vi "Procesado_aRMS_BIdirecc.vi"(0 "Paths_canales_aRMS":path[](array[path]), 3 "Ejes Procesados":i32, 4 "Distancias\nacelerometros":dbl[](array[numeric]), 6 "Distancias generales (m)":dbl[](array[numeric]), 7 "Distancias centrales de las ruedas\n               configuración (m)":dbl[](array[numeric]), 8 "Frecuencia de muestreo":dbl, 9 "Parámetros acelerómetros":dbl[](array[numeric]), 10 "dt RMS 2":dbl, 11 "Puntos":sgl[](array[numeric])) -> (1 "Max RMS Ruedas":dbl[][](array[numeric]))   [LabVIEW 2015]
uses:
  <vilib>/Analysis/3filter.llb/Filter Passband Type.ctl
  <vilib>/Analysis/5stat.llb/RMS (DBL).vi
  <vilib>/Analysis/3filter.llb/Butterworth Filter (DBL).vi
  <vilib>/measure/madcrms.llb/Basic Averaged DC-RMS for 1 Chan.vi
  <vilib>/measure/NI_MAPro.lvlib
  <vilib>/Analysis/NI_AALBase.lvlib
  <vilib>/Analysis/NI_AALPro.lvlib
panel:
  out "Array 2":dbl[][](array[numeric])
  out "Array":dbl[][](array[numeric])
  out "Loop Rate (Hz)":dbl
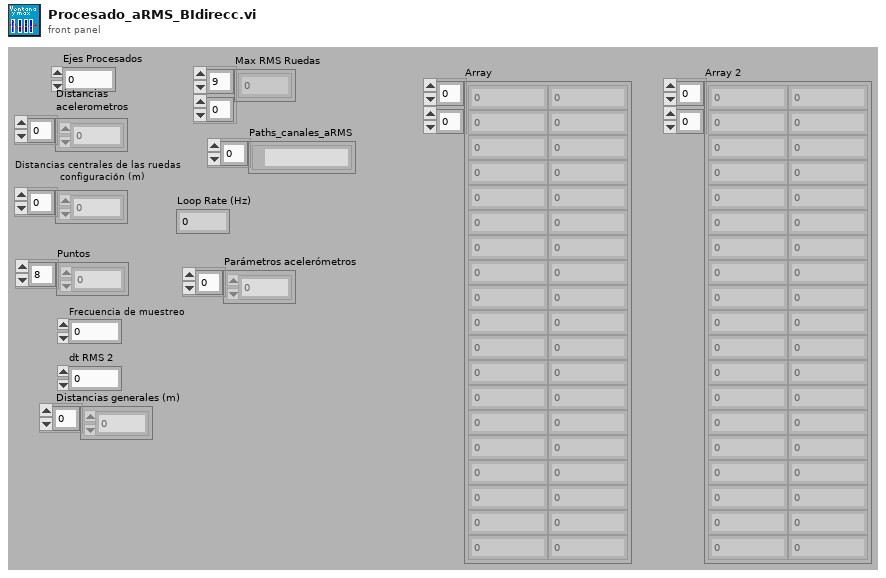
[diagram p1: front panel]
types:
  T1 = typedef "NI_AALBase.lvlib/Filter Passband Type.ctl" = enum32{"Lowpass", "Highpass", "Bandpass", "Bandstop"}
  T2 = enum16{"big-endian, network order", "native, host order", "little-endian"}
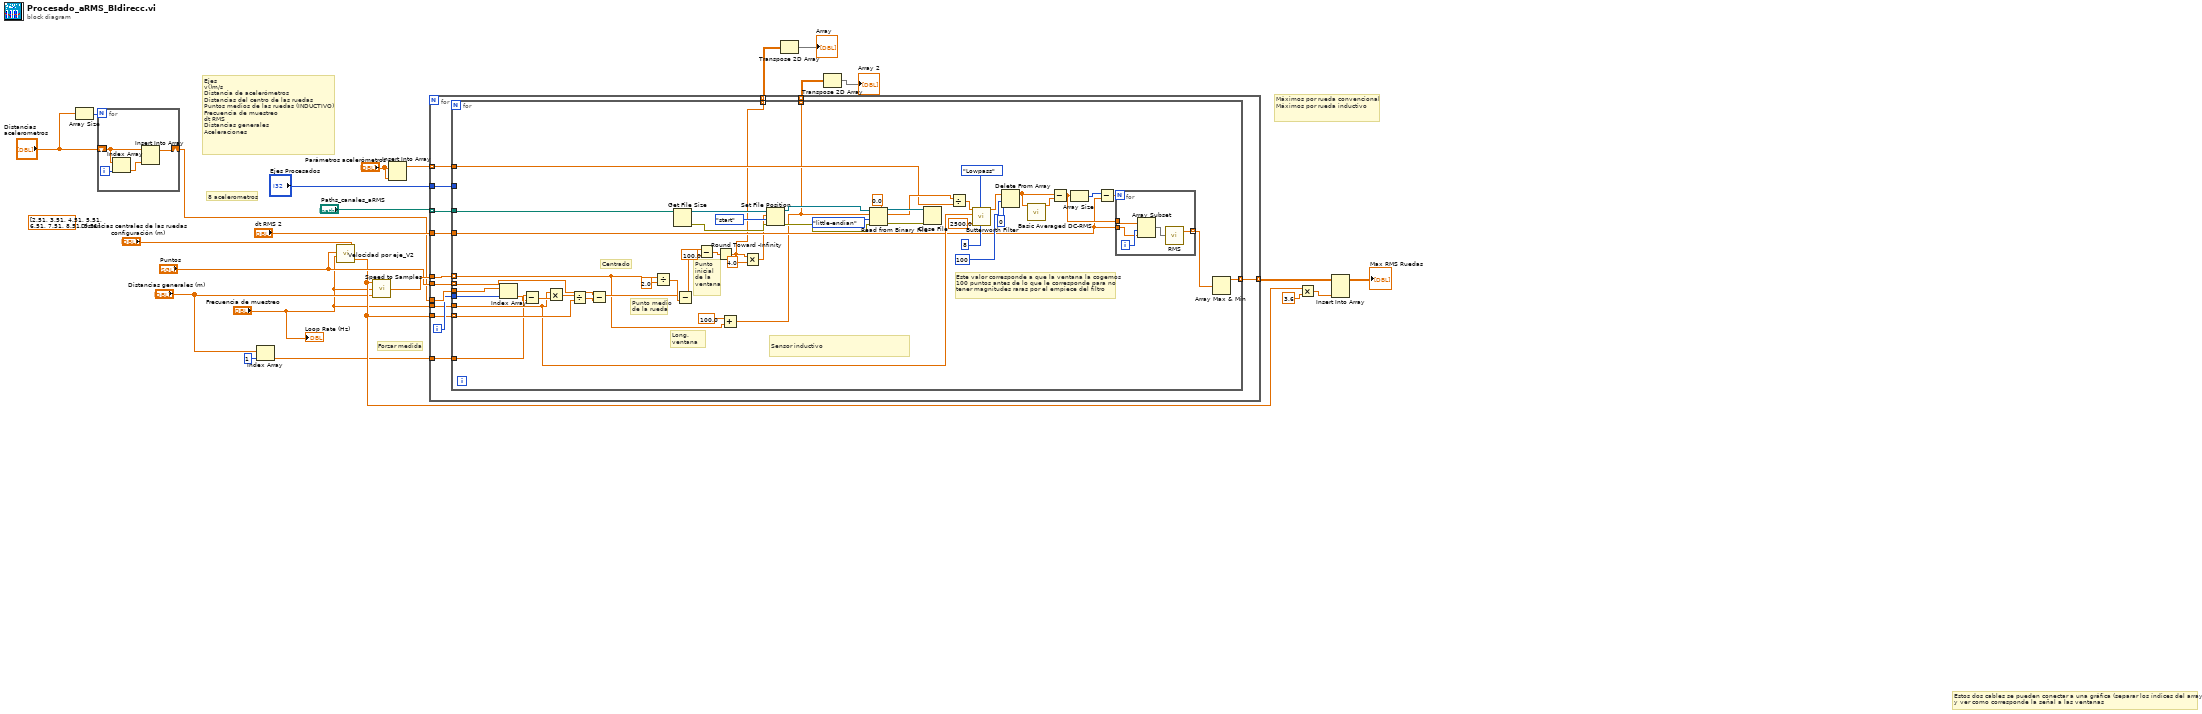
[diagram p0: block diagram]
diagram:
  (unwired) dbl[] [2.51, 3.51, 4.51, 5.51, 6.51, 7.51, 8.51, 9.51] ("Distancias\nacelerometros")
  # "Forzar medida"
  # "8 acelerometros"
  # "Ejes\nv()m/s\nDistancia de acelerómetros\nDistancias del centro de las ruedas\nPuntos medios de las ruedas (INDUCTIVO)\nFrecuencia de muestreo\ndt RMS\nDistancias generales\nAceleraciones"
  # "Máximos por rueda convencional\nMáximos por rueda inductivo"
  # "Estos dos cables se pueden conectar a una gráfica (separar los índices del array)\ny ver como corresponde la señal a las ventanas"
  n1 = Array Size(array="Distancias\nacelerometros") -> (size(s)=w8:i32)
  n2 = for {
    N: w8 -> [_]
    shift-right: [w28] -> w2
    shift-left: "Distancias\nacelerometros" -> [w27]
    i -> [w26]
    n3 = Index Array(array=w27, index=w26) -> (element=w25:dbl)
    n4 = Insert Into Array(array=w27, new element=w25) -> (w28:dbl[])  [unwired: 1 in]
  }
  n5 = Index Array(array="Distancias generales (m)", index=1) -> (element=w1:dbl)
  n6 = call "Velocidad por eje_V2.vi"("Distancias centrales de las ruedas\n               configuración (m)"="Distancias centrales de las ruedas\n               configuración (m)", "Frecuencia de muestreo"="Frecuencia de muestreo", "Puntos centrales de las ruedas\n             inductivo"="Puntos") -> ("Velocidad de eje"=w18:dbl[])  [unwired: 2 in]
  n7 = call "Speed to Samples.vi"("Distancias generales (m)"="Distancias generales (m)", "Loop Rate (Hz)"="Frecuencia de muestreo", "Velocidad de eje(m/s)"=w18) -> ("Longitud de ventana (puntos)"=w24:dbl[])
  n8 = Insert Into Array(array="Parámetros acelerómetros", new element="Parámetros acelerómetros") -> (w13:dbl[])  [unwired: 1 in]
  n9 = for {
    tunnel: w24 -> [w32]
    tunnel: "Puntos" -> [w40]
    tunnel: w18 -> [w37]
    tunnel: w2 -> [w41]
    tunnel: "dt RMS 2" -> [w42]
    tunnel: [w39] -> w20 mode=indexing
    tunnel: "Ejes Procesados" -> [w33]
    tunnel: "Frecuencia de muestreo" -> [w34]
    tunnel: "Paths_canales_aRMS" -> [w36] mode=indexing
    tunnel: w13 -> [w35] mode=indexing
    tunnel: w1 -> [w31]
    tunnel: [w30] -> w3 mode=indexing
    tunnel: [w29] -> w6 mode=indexing
    i -> [w38]
    n10 = for {
      tunnel: w42 -> [w49]
      tunnel: w41 -> [w90]
      tunnel: w40 -> [w89] mode=indexing
      tunnel: [w88] -> w39 mode=indexing
      tunnel: w38 -> [w87]
      tunnel: w37 -> [w86] mode=indexing
      tunnel: w36 -> [w71]
      tunnel: w35 -> [w80]
      tunnel: w34 -> [w63]
      tunnel: w33 -> [_]
      tunnel: w32 -> [w60] mode=indexing
      tunnel: w31 -> [w47]
      tunnel: [w44] -> w30 mode=indexing
      tunnel: [w43] -> w29 mode=indexing
      # "Este valor corresponde a que la ventana la cogemos\n100 puntos antes de lo que le corresponde para no \ntener magnitudes raras por el empiece del filtro"
      # "Centrado"
      # "Sensor inductivo"
      # "Long.\nventana"
      # "Punto\ninicial\nde la \nventana"
      # "Punto medio\nde la rueda"
      n11 = Index Array(array=w90, index=w87) -> (element=w46:dbl)
      n12 = Subtract(x=w47, y=w46) -> (x-y=w74:dbl)
      n13 = Multiply(x=w63, y=w74) -> (x*y=w76:dbl)
      n14 = Divide(x=w76, y=w86) -> (x/y=w75:dbl)
      n15 = Subtract(x=w89, y=w75) -> (x-y=w64:dbl)
      n16 = Divide(x=w60, y=2.0) -> (x/y=w72:dbl)
      n17 = Get File Size(file=w71) -> (refnum out=w69:refnum<file>, 0:w66:errorcluster)  [unwired: 1 in, 1 out]
      n18 = Subtract(x=w64, y=w72) -> (x-y=w54:dbl)
      n19 = Subtract(x=w54, y=100.0 ("x")) -> (x-y=w62:dbl)
      n20 = Round Toward -Infinity(1:w62) -> (0:w44:dbl)
      n21 = Add(x=100.0, y=w60) -> (x+y=w43:dbl)
      n22 = Multiply(x=w44, y=4.0) -> (x*y=w45:dbl)
      n23 = Set File Position(offset (in bytes) (0)=w45, refnum=w69, from (0:start)=enum16{"start", "end", "current"}."start", error in=w66) -> (refnum out=w67:refnum<file>, error out=w65:errorcluster)
      n24 = Read from Binary File(5:sgl 0.0, 8:w65, 9:T2."little-endian" ("byte order (0:big-endian, network order)"), 10:w43, 11:w67) -> (0:w84:errorcluster, 2:w81:sgl[], 3:w85:refnum<file>)  [unwired: 2 out]
      n25 = Close File(refnum=w85, error in=w84) -> ()  [unwired: 2 out]
      n26 = Divide(x=w81, y=w80) -> (x/y=w77:dbl[])
      n27 = call-poly <vilib>:"Butterworth Filter.vi"("order"=8, "filter type"=Filter_Passband_Type."Lowpass", "low cutoff freq: fl"=2500.0, "sampling freq: fs"=w63, "X"=w77) -> ("Filtered X"=w59:dbl[])  [unwired: 3 in, 1 out]
      n28 = Delete From Array(array=w59, length=100, index=0) -> (array with subset deleted=w58:dbl[])  [unwired: 1 out]
      n29 = call-poly <vilib>:"Basic Averaged DC-RMS.vi"("signal in"=w58) -> ("DC value"=w91:dbl)  [unwired: 4 in, 6 out]
      n30 = Subtract(x=w58, y=w91) -> (x-y=w52:dbl[])
      n31 = Array Size(array=w52) -> (size(s)=w50:i32)
      n32 = Subtract(x=w50, y=w49) -> (x-y=w51:dbl)
      n33 = for {
        N: w51 -> [_]
        tunnel: w49 -> [w93]
        tunnel: [w96] -> w48 mode=indexing
        tunnel: w52 -> [w95]
        i -> [w94]
        n34 = Array Subset(array=w95, index=w94, length=w93) -> (w92:dbl[])
        n35 = call-poly <vilib>:"RMS.vi"("X"=w92) -> ("rms value"=w96:dbl)  [unwired: 1 out]
      }
      n36 = Array Max & Min(array=w48) -> (max value=w88:dbl)  [unwired: 3 out]
    }
  }
  n37 = Transpose 2D Array(2D array=w3) -> (transposed array=→"Array":dbl[][])
  n38 = Transpose 2D Array(2D array=w6) -> (transposed array=→"Array 2":dbl[][])
  n39 = Multiply(x=w18, y=3.6) -> (x*y=w16:dbl[])
  n40 = Insert Into Array(array=w20, new element=w16) -> (→"Max RMS Ruedas":dbl[][])  [unwired: 2 in]
  "Loop Rate (Hz)" <- "Frecuencia de muestreo"
